vi "Write Left Joystick.vi"(8 "error in (no error)":errorcluster, 10 "XBoxJoystick":T1 {"Right" scale=-1.0..1.0; "Forward" scale=-1.0..1.0}, 11 "XBoxController in":refnum<class "XBoxController.lvclass">) -> (0 "error out":errorcluster, 3 "XBoxController out":refnum<class "XBoxController.lvclass">)   [LabVIEW 2013, in "XBoxController.lvclass"]
uses:
  XBoxController.lvclass
  XBoxJoystick.ctl
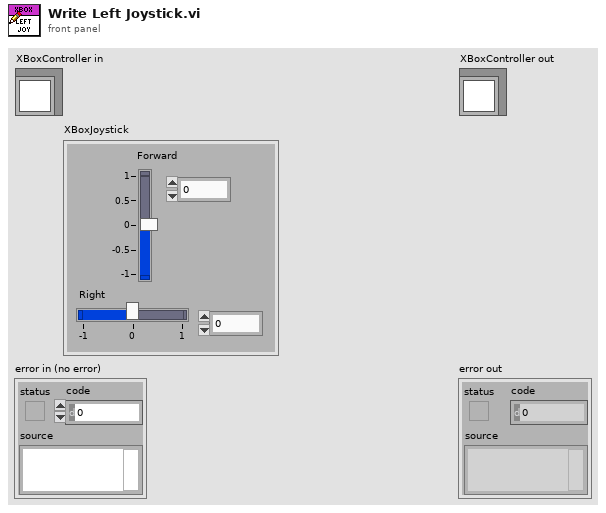
[diagram p1: front panel]
types:
  T1 = typedef "XBoxController.lvclass/XBoxJoystick.ctl" = cluster{"Forward":dbl, "Right":dbl}
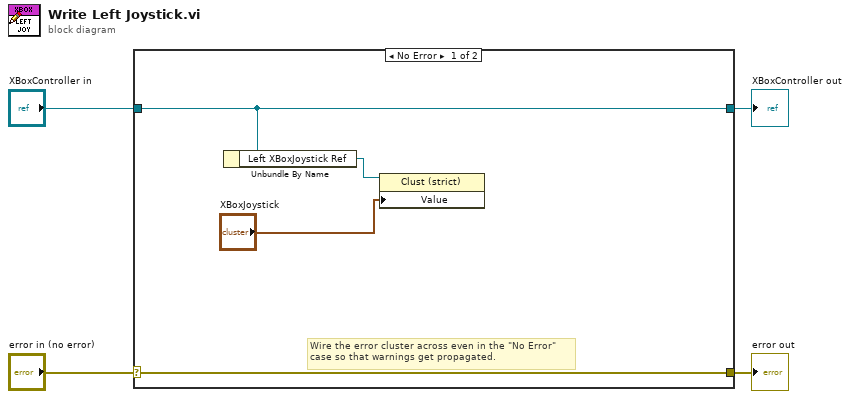
[diagram p0: block diagram]
diagram:
  n1 = case shown="No Error" "error in (no error)" {
    selector: "error in (no error)" -> [w8 w10]
    tunnel: [w8 w10] -> w3
    tunnel: [w7 w9] -> w1
    tunnel: "XBoxController in" -> [w7 w9]
    frame No Error {
      # "Wire the error cluster across even in the \"No Error\"\ncase so that warnings get propagated."
      n2 = Unbundle By Name(w7) -> ("Left XBoxJoystick Ref"=w6:refnum<vi>)
      n3 = property class="Clust (strict)"(reference=w6, "Value"="XBoxJoystick") -> ()  [unwired: 1 in, 2 out]
    }
    frame Error {
    }
  }
  "error out" <- w3
  "XBoxController out" <- w1
